vi "Simulate_Task.vi"(9 "DeamonQueueName":string, 11 "Parent VI":refnum<vi>) -> ()   [LabVIEW 2024]
doc: "Program symulujący działanie piekarnika z 2 grzałkami i wentylatorem, konfigurowalny przy pomocy pliku .txt. Symulacja odbywa się co 100ms, do komunikacji z programem służą funkcje: set_Heaters, set_Fan i get_Temperature."
uses:
  TypeDefs/Heater_interface.ctl
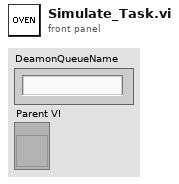
[diagram p1: front panel]
types:
  T1 = typedef "Heater_interface.ctl" = enum16{"setSpeed", "setHeaters", "getTemperature"}
  T2 = cluster{"Actions\n":T1, "Parameter1":variant, "Parameter2\n":variant}
  T3 = cluster{"Heater1":dbl, "Heater2\n":dbl, "Fan":dbl, "Temperature":dbl, "EN_HEATER1":dbl, "EN_HEATER2":dbl, "EN_FAN":dbl}
  T4 = enum16{"open", "replace", "create", "open or create", "replace or create", "replace or create with confirmation"}
  T5 = enum32{"Bad", "Idle", "Run top level", "Running"}
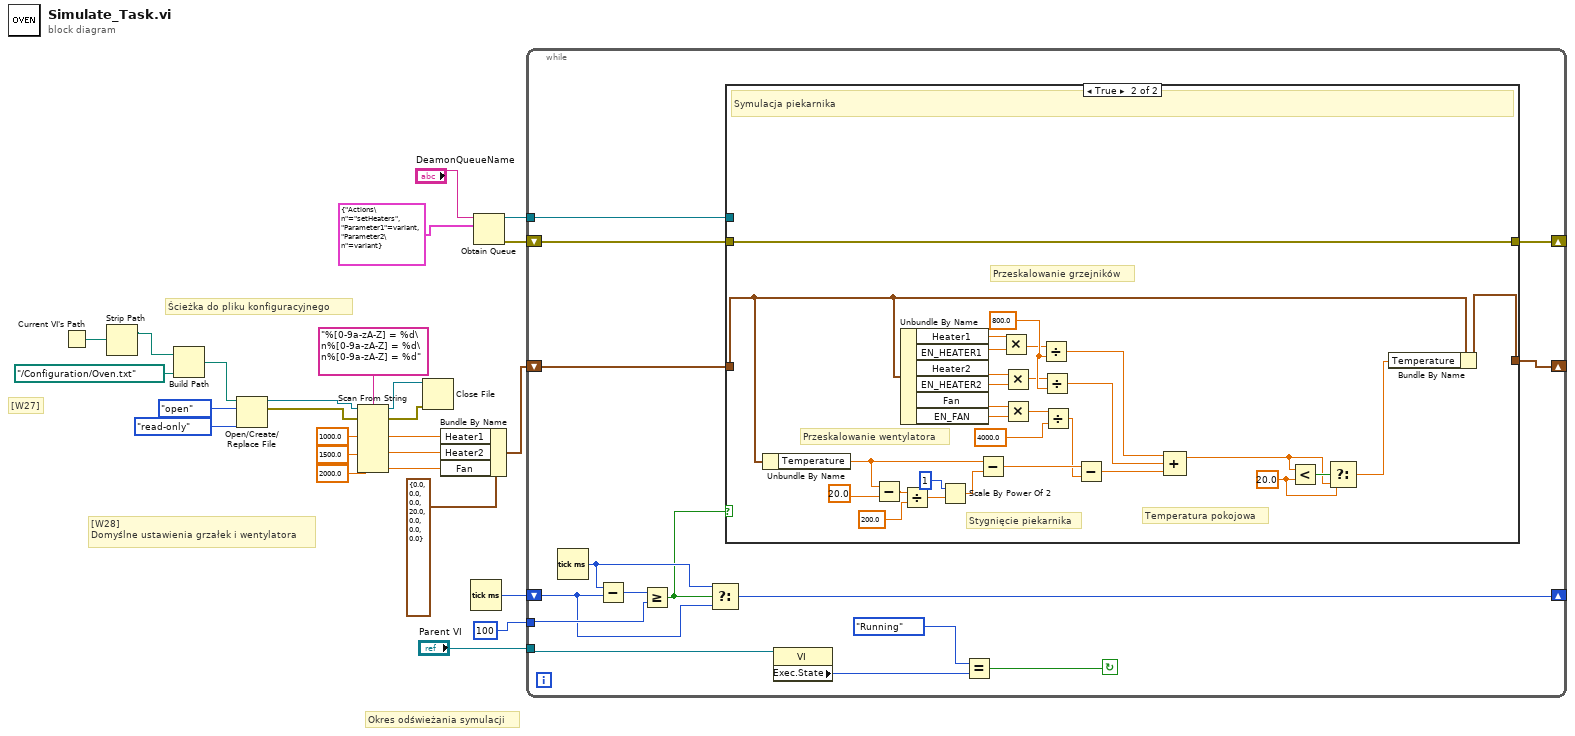
[diagram p0: block diagram]
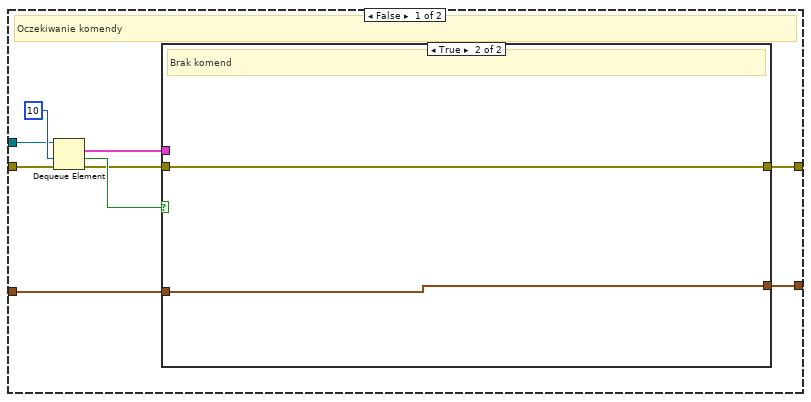
[diagram p2: hidden frame]
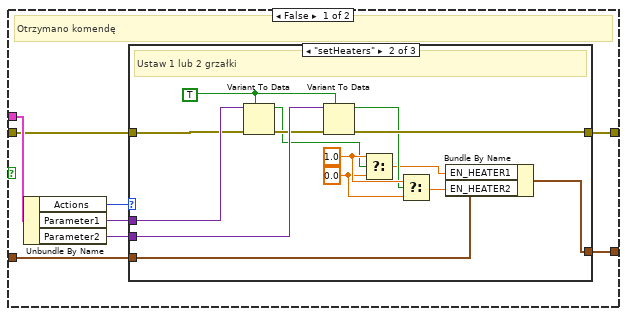
[diagram p3: hidden frame]
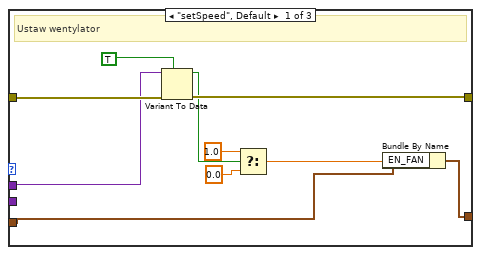
[diagram p4: hidden frame]
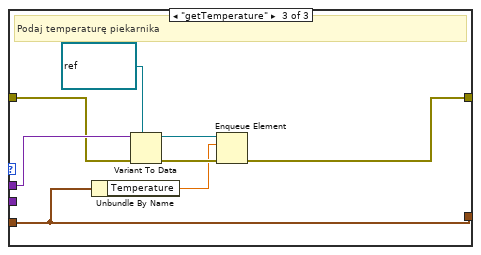
[diagram p5: hidden frame]
diagram:
  # "[W27]"
  # "Okres odświeżania symulacji"
  # "[W28]\nDomyślne ustawienia grzałek i wentylatora"
  # "Ścieżka do pliku konfiguracyjnego"
  n1 = Current VI's Path() -> (path=w14:path)
  n2 = Strip Path(path=w14) -> (stripped path=w13:path)  [unwired: 1 out]
  n3 = Build Path(base path=w13, name or relative path=path "../Configuration/Oven.txt") -> (appended path=w15:path)
  n4 = Open/Create/Replace File(file path (use dialog)=w15, operation (0:open)=T4."open", access (0:read/write)=enum16{"read/write", "read-only", "write-only"}."read-only") -> (refnum out=w24:refnum<file>, error out=w23:errorcluster)  [unwired: 3 in, 1 out]
  n5 = Scan From String("%[0-9a-zA-Z] = %d\n%[0-9a-zA-Z] = %d\n%[0-9a-zA-Z] = %d" ("prompt"), w24, w23, default 2=1000.0 ("default value 2"), default 4=1500.0 ("default value 4"), default 6=2000.0 ("default value 6")) -> (w22:refnum<file>, w21:errorcluster, output 2=w11:dbl, output 4=w10:dbl, output 6=w9:dbl)  [unwired: 6 in]
  n6 = Close File(refnum=w22, error in=w21) -> ()  [unwired: 2 out]
  n7 = Bundle By Name(cluster=T3 {"Heater1"=0.0, "Heater2\n"=0.0, "Fan"=0.0, "Temperature"=20.0, "EN_HEATER1"=0.0, "EN_HEATER2"=0.0, "EN_FAN"=0.0}, "Heater1"=w11, "Heater2"=w10, "Fan"=w9) -> (w8:T3)
  n8 = Tick Count (ms)() -> (millisecond timer value=w1:u32)
  n9 = Obtain Queue(name (unnamed)="DeamonQueueName", element data type=T2 {"Actions\n"=enum."setHeaters", "Parameter1"=variant, "Parameter2\n"=variant}) -> (queue out=w5:refnum<queue>, error out=w4:errorcluster)  [unwired: 3 in, 1 out]
  n10 = while {
    shift-right: [w37] -> _
    shift-left: w8 -> [w38]
    tunnel: w5 -> [w40]
    shift-right: [w39] -> _
    shift-left: w4 -> [w41]
    tunnel: "Parent VI" -> [w28]
    tunnel: u32 100 ("y") -> [w33]
    shift-right: [w27] -> _
    shift-left: w1 -> [w32]
    stop <- w29 continue-if-true
    n11 = Tick Count (ms)() -> (millisecond timer value=w36:u32)
    n12 = Subtract(x=w36, y=w32) -> (x-y=w35:u32)
    n13 = Greater Or Equal?(x=w35, y=w33) -> (x >= y?=w34:bool)
    n14 = Select(t=w36, s=w34, f=w32) -> (s? t:f=w27:u32)
    n15 = case shown="True" w34 {
      tunnel: w41 -> [w49 w122]
      tunnel: w40 -> [w48 _]
      tunnel: [w44 w122] -> w39
      tunnel: w38 -> [w43 w120]
      tunnel: [w42 w121] -> w37
      frame False {
        # "Oczekiwanie komendy"
        n16 = Dequeue Element(queue=w48, timeout in ms (-1)=10, error in (no error)=w49) -> (element=w46:T2, timed out?=w47:bool, error out=w45:errorcluster)  [unwired: 1 out]
        n17 = case shown="True" w47 {
          tunnel: w46 -> [w58 _]
          tunnel: w45 -> [w55 w92]
          tunnel: [w54 w92] -> w44
          tunnel: w43 -> [w53 w91]
          tunnel: [w52 w91] -> w42
          frame False {
            # "Otrzymano komendę"
            n18 = Unbundle By Name(w58) -> ("Actions"=w57:T1, "Parameter1"=w56:variant, "Parameter2"=w51:variant)
            n19 = case shown="\"setHeaters\"" w57 {
              tunnel: w56 -> [w66 w82 w87]
              tunnel: w55 -> [w68 w81 w86]
              tunnel: [w67 w76 w85] -> w54
              tunnel: w53 -> [w61 w80 w84]
              tunnel: [w65 w79 w84] -> w52
              tunnel: w51 -> [_ w78 _]
              frame "setSpeed", Default {
                # "Ustaw wentylator"
                n20 = Variant To Data(error in=w68, type=TRUE ("Boolean"), Variant=w66) -> (data=w63:bool, error out=w67:errorcluster)
                n21 = Select(t=1.0 ("f"), s=w63, f=0.0) -> (s? t:f=w60:dbl)
                n22 = Bundle By Name(cluster=w61, "EN_FAN"=w60) -> (w65:T3)
              }
              frame "setHeaters" {
                w73 = 0.0
                w74 = 1.0 ("t")
                w75 = TRUE ("Boolean")
                # "Ustaw 1 lub 2 grzałki"
                n23 = Variant To Data(error in=w81, type=w75, Variant=w82) -> (data=w72:bool, error out=w77:errorcluster)
                n24 = Variant To Data(error in=w77, type=w75, Variant=w78) -> (data=w71:bool, error out=w76:errorcluster)
                n25 = Select(t=w74, s=w72, f=w73) -> (s? t:f=w70:dbl)
                n26 = Select(t=w74, s=w71, f=w73) -> (s? t:f=w69:dbl)
                n27 = Bundle By Name(cluster=w80, "EN_HEATER1"=w70, "EN_HEATER2"=w69) -> (w79:T3)
              }
              frame "getTemperature" {
                # "Podaj temperaturę piekarnika"
                n28 = Unbundle By Name(w84) -> ("Temperature"=w83:dbl)
                n29 = Variant To Data(error in=w86, type=refnum<queue> refnum ("queue out"), Variant=w87) -> (data=w89:refnum<queue>, error out=w88:errorcluster)
                n30 = Enqueue Element(queue=w89, element=w83, error in (no error)=w88) -> (error out=w85:errorcluster)  [unwired: 1 in, 2 out]
              }
            }
          }
          frame True {
            # "Brak komend"
          }
        }
      }
      frame True {
        w100 = 800.0
        w111 = 20.0 ("y")
        # "Stygnięcie piekarnika"
        # "Przeskalowanie wentylatora"
        # "Przeskalowanie grzejników"
        # "Temperatura pokojowa"
        # "Symulacja piekarnika"
        n31 = Unbundle By Name(w120) -> ("Temperature"=w105:dbl)
        n32 = Subtract(x=w105, y=20.0) -> (x-y=w107:dbl)
        n33 = Unbundle By Name(w120) -> ("Heater1"=w119:dbl, "EN_HEATER1"=w118:dbl, "Heater2"=w117:dbl, "EN_HEATER2"=w116:dbl, "Fan"=w115:dbl, "EN_FAN"=w114:dbl)
        n34 = Divide(x=w107, y=200.0) -> (x/y=w102:dbl)
        n35 = Scale By Power Of 2(n=i16 1, x=w102) -> (x*2^n=w101:dbl)
        n36 = Subtract(x=w105, y=w101) -> (x-y=w108:dbl)
        n37 = Multiply(x=w119, y=w118) -> (x*y=w97:dbl)
        n38 = Multiply(x=w117, y=w116) -> (x*y=w99:dbl)
        n39 = Multiply(x=w115, y=w114) -> (x*y=w98:dbl)
        n40 = Divide(x=w97, y=w100) -> (x/y=w96:dbl)
        n41 = Divide(x=w99, y=w100) -> (x/y=w95:dbl)
        n42 = Divide(x=w98, y=4000.0) -> (x/y=w94:dbl)
        n43 = Subtract(x=w108, y=w94) -> (x-y=w113:dbl)
        n44 = Compound Arithmetic op=ADD(w96, w95, w113) -> (w110:dbl)
        n45 = Less?(x=w110, y=w111) -> (x < y?=w112:bool)
        n46 = Select(t=w111, s=w112, f=w110) -> (s? t:f=w109:dbl)
        n47 = Bundle By Name(cluster=w120, "Temperature"=w109) -> (w121:T3)
      }
    }
    n48 = property class="VI"(reference=w28) -> ("Exec.State"=w31:T5)  [unwired: 1 in, 2 out]
    n49 = Equal?(x=T5."Running", y=w31) -> (x = y?=w29:bool)
  }
